vi "HideGroup.vi"(8 "error in (no error)":errorcluster, 9 "GroupCol Index":i32=3, 10 "String toHide":string, 11 "Table CtlRef In":refnum<vi>) -> (0 "error out":errorcluster, 3 "Table CtlRef Out":refnum<vi>)   [LabVIEW 2013]
doc: "Searches table data in GroupCol for \"String toHide,\" setting row height to zero if it matches."
uses:
  <vilib>/Utility/miscctls.llb/LVRowAndColumnTypeDef.ctl
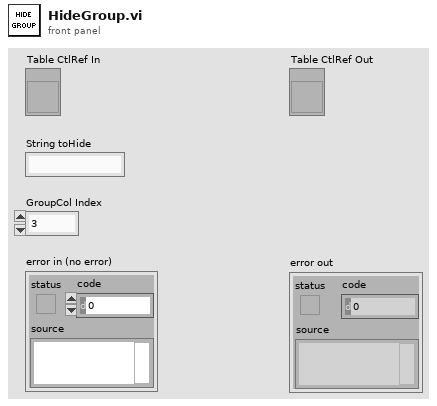
[diagram p1: front panel]
types:
  T1 = typedef "LVRowAndColumnTypeDef.ctl" = cluster{"Row":i32, "Column":i32}
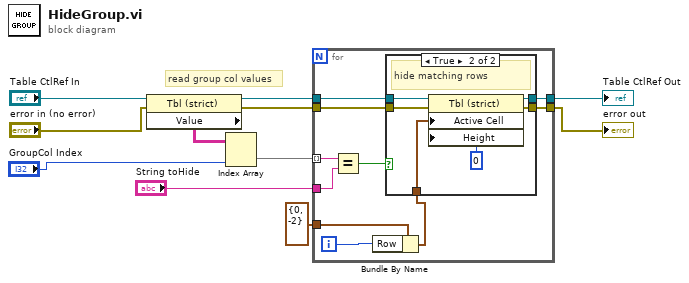
[diagram p0: block diagram]
diagram:
  # "read group col values"
  n1 = property class="Tbl (strict)"(reference="Table CtlRef In", error in="error in (no error)") -> (reference out=w8:refnum<vi>, error out=w9:errorcluster, "Value"=w10:string[][])
  n2 = Index Array(array=w10, index (col)="GroupCol Index") -> (element=w11:string[])  [unwired: 1 in]
  n3 = for {
    tunnel: w8 -> [w21]
    tunnel: w9 -> [w20]
    tunnel: [w19] -> w4
    tunnel: [w18] -> w5
    tunnel: w11 -> [w14] mode=indexing
    tunnel: T1 {"Row"=0, "Column"=-2} ("Cell Position") -> [w16]
    tunnel: "String toHide" -> [w13]
    i -> [w17]
    n4 = Equal?(x=w14, y=w13) -> (x = y?=w12:bool)
    n5 = Bundle By Name(cluster=w16, "Row"=w17) -> (w15:T1)
    n6 = case shown="True" w12 {
      tunnel: w21 -> [w23 w29]
      tunnel: w20 -> [w22 w28]
      tunnel: [w22 w27] -> w19
      tunnel: [w23 w26] -> w18
      tunnel: w15 -> [_ w24]
      frame False {
      }
      frame True {
        # "hide matching rows"
        n7 = property class="Tbl (strict)"(reference=w29, error in=w28, "Active Cell"=w24, "Height"=u32 0 ("Active Cell:Cell Size:Height")) -> (reference out=w26:refnum<vi>, error out=w27:errorcluster)
      }
    }
  }
  "error out" <- w4
  "Table CtlRef Out" <- w5
